vi "Main.vi"() -> ()   [LabVIEW 2019, in "gRPC Template Creation Utility.lvlib"]
uses:
  gRPC Template Creation Utility.lvlib
  TypeDefs/Project Settings.ctl
panel:
  in  "Library Suffix":string caption="Generated Library Suffix (\"_server\" / \"_client\" will be auto appended by default)"
  in  "Proto File Path":path[](array[path])
  in  "Generate":enum16{"gRPC Server", "gRPC Client", "Both"}(ring)
  in  "Target Name":string
  in  "Generated Library Name":string
  in  "Target Project":path
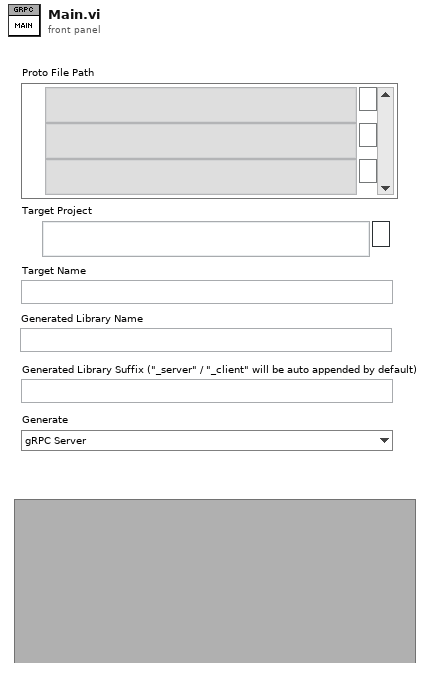
[diagram p1: front panel]
types:
  T1 = typedef "gRPC Template Creation Utility.lvlib/RPC Method Parameters.ctl" = cluster{"RPC Method Name":string, "Request Metadata Name":string, "Response Metadata Name":string, "Client Streaming":bool, "Server Streaming":bool}
  T2 = typedef "gRPC Template Creation Utility.lvlib/Message Metadata (Scripting).ctl" = cluster{"Version":i32, "Name":string, "Type Url":string, "Elements":T3[]}
  T3 = typedef "gRPC Template Creation Utility.lvlib/Message Element Metadata (Scripting).ctl" = cluster{"Field Name":string, "Embedded Message Name":string, "Protobuf Index":i32, "MessageElementType":T4, "Repeated":bool}
  T4 = typedef "gRPC Template Creation Utility.lvlib/Message Element Type.ctl" = enum32{"Int32Value", "FloatValue", "DoubleValue", "BoolValue", "StringValue", "MessageValue", "Int64Value", "UInt32Value", "UInt64Value", "EnumValue", "Bytes", "Fixed64", "Fixed32", "SFixed64", "SFixed32", "SInt64", "SInt32"}
  T5 = typedef "gRPC Template Creation Utility.lvlib/Project Settings.ctl" = cluster{"Target Project Path":path, "Target Name":string, "Server Name":string, "Library Path":path}
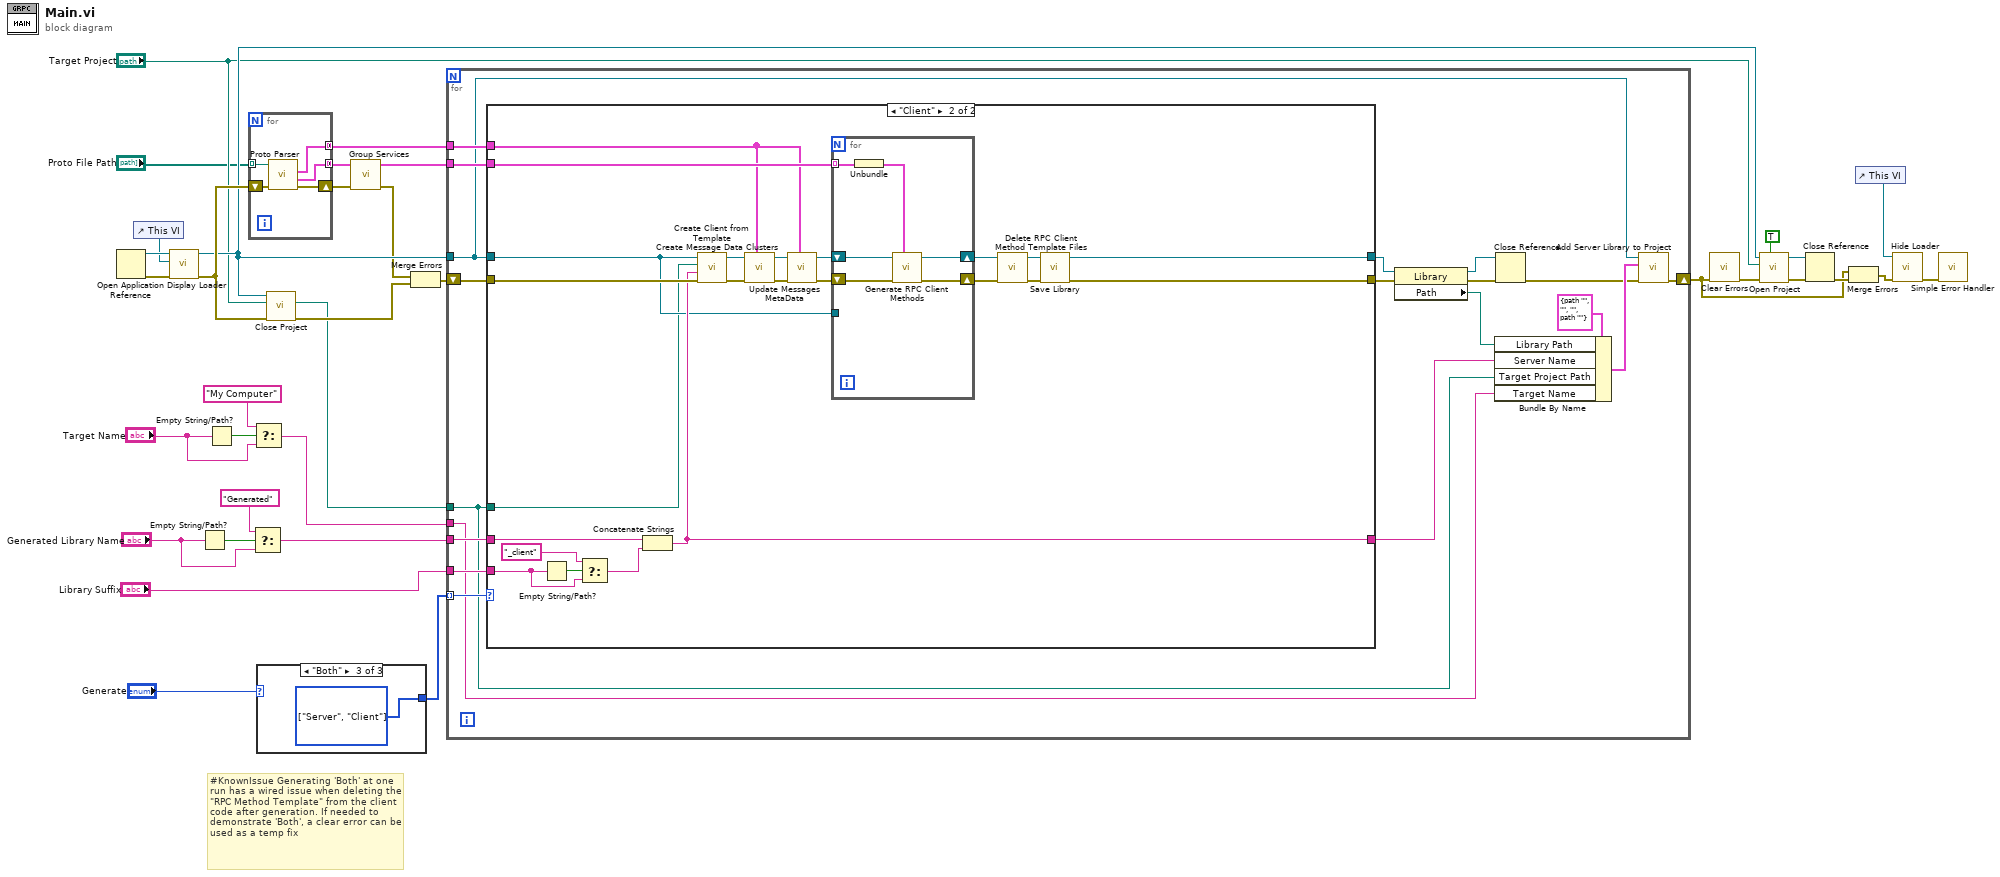
[diagram p0: block diagram]
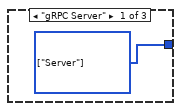
[diagram p2: hidden frame]
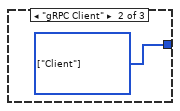
[diagram p3: hidden frame]
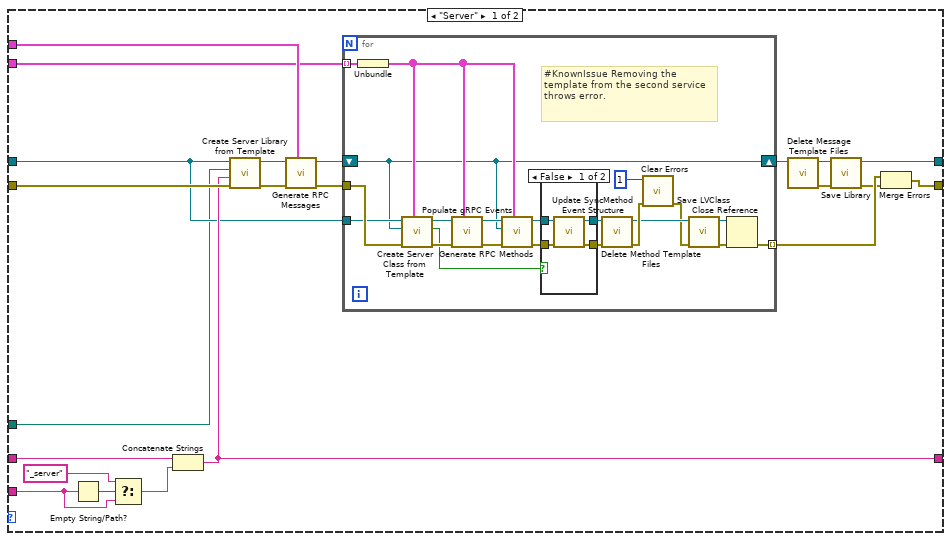
[diagram p4: hidden frame]
diagram:
  # "#KnownIssue Generating 'Both' at one run has a wired issue when deleting the \"RPC Method Template\" from the client code after generation. If needed to demonstrate 'Both', a clear error can be used as a temp fix"
  n1 = Open Application Reference() -> (0:w28:errorcluster, 3:w27:refnum<vi>)  [unwired: 4 in]
  n2 = control-ref of="This VI"() -> (w25:refnum<vi>)
  n3 = call "Display Loader.vi"("error in (no error)"=w28, "VI in"=w25, "application ref in"=w27) -> ("error out"=w26:errorcluster, "application ref out"=w13:refnum<vi>)  [unwired: 7 in]
  n4 = Empty String/Path?(string/path="Generated Library Name") -> (empty?=w35:bool)
  n5 = Empty String/Path?(string/path="Target Name") -> (empty?=w20:bool)
  n6 = for {
    tunnel: [w39] -> w30 mode=concatenating
    tunnel: [w38] -> w3 mode=concatenating
    shift-right: [w40] -> w5
    shift-left: w26 -> [w37]
    tunnel: "Proto File Path" -> [w36] mode=indexing
    n7 = call "Proto Parser.vi"("error in (no error)"=w37, ".proto file path"=w36) -> ("error out"=w40:errorcluster, "gRPC Method Parameters"=w38:T1[], "gRPC Messages Parameters"=w39:T2[])  [unwired: 7 in]
  }
  n8 = Select(t="Generated" ("Path"), s=w35, f="Generated Library Name") -> (s? t:f=w22:string)
  n9 = Select(t="My Computer" ("Path"), s=w20, f="Target Name") -> (s? t:f=w18:string)
  n10 = case shown="\"Both\"" "Generate" {
    tunnel: [w41 w42 w43] -> w17
    frame "gRPC Server" {
      w41 = enum16{"Server", "Client"}[] [enum."Server"] items=["Server", "Client"]
    }
    frame "gRPC Client" {
      w42 = enum16{"Server", "Client"}[] [enum."Client"] items=["Server", "Client"]
    }
    frame "Both" {
      w43 = enum16{"Server", "Client"}[] [enum."Server", enum."Client"] items=["Server", "Client"]
    }
  }
  n11 = call "Close Project.vi"("error in (no error)"=w26, "Project Path in"="Target Project", "Application reference"=w13) -> ("error out"=w32:errorcluster, "Project Path out"=w23:path)  [unwired: 6 in, 1 out]
  n12 = call "Group Services.vi"("error in"=w5, "gRPC Method Parameters"=w3) -> ("error out"=w4:errorcluster, "Service Methods"=w2:cluster{"gRPC Method Parameters":T1[]}[])  [unwired: 8 in]
  n13 = Merge Errors(w4, w32) -> (w31:errorcluster)
  n14 = for {
    tunnel: w30 -> [w61]
    tunnel: w2 -> [w60]
    tunnel: w23 -> [w45]
    tunnel: w22 -> [w53]
    tunnel: w18 -> [w44]
    tunnel: w13 -> [w51]
    shift-right: [w48] -> w7
    shift-left: w31 -> [w62]
    tunnel: w17 -> [w47] mode=indexing
    tunnel: "Library Suffix" -> [w46]
    n15 = case shown="\"Client\"" w47 {
      tunnel: w62 -> [w84 w134]
      tunnel: w61 -> [w83 w123]
      tunnel: w60 -> [w82 w133]
      tunnel: [w81 w132] -> w59
      tunnel: [w80 w120] -> w57
      tunnel: w53 -> [w79 w131]
      tunnel: [w78 w130] -> w52
      tunnel: w51 -> [w77 w129]
      tunnel: w45 -> [w76 w128]
      tunnel: w46 -> [w63 w113]
      frame "Server" {
        n16 = Empty String/Path?(string/path=w63) -> (empty?=w66:bool)
        n17 = Select(t="_server" ("string"), s=w66, f=w63) -> (s? t:f=w64:string)
        n18 = Concatenate Strings(w79, w64) -> (w78:string)
        n19 = call "Create Server Library from Template.vi"("error in (no error)"=w84, "Generated Server Name"=w78, "Target Project Path"=w76, "Application ref in"=w77) -> ("error out"=w74:errorcluster, "Server library out"=w75:refnum<vi>)  [unwired: 6 in]
        n20 = call "Generate RPC Messages.vi"("Messages MetaData"=w83, "error in (no error)"=w74, "Library"=w75) -> ("error out"=w72:errorcluster, "Library"=w73:refnum<vi>)  [unwired: 7 in]
        n21 = for {
          tunnel: w82 -> [w103] mode=indexing
          shift-right: [w94] -> w71
          shift-left: w73 -> [w94]
          tunnel: w77 -> [w104]
          tunnel: w72 -> [w105]
          tunnel: [w100] -> w70 mode=indexing
          # "#KnownIssue Removing the template from the second service throws error."
          n22 = Unbundle(w103) -> ("gRPC Method Parameters"=w95:T1[])
          n23 = call "Create Server Class from Template.vi"("gRPC Method Parameters"=w95, "error in (no error)"=w105, "Library"=w94, "Application ref in"=w104) -> ("error out"=w98:errorcluster, "Already Exists ?"=w89:bool, "LVClassLibrary in"=w99:refnum<vi>)  [unwired: 5 in]
          n24 = call "Populate gRPC Events.vi"("RPC Method Parameters"=w95, "error in (no error)"=w98, "Server class in"=w99) -> ("error out"=w96:errorcluster, "Server class out"=w97:refnum<vi>)  [unwired: 7 in]
          n25 = call "Generate RPC Methods.vi"("RPC Method Parameters"=w95, "error in (no error)"=w96, "Library"=w94, "Server class in"=w97) -> ("error out"=w91:errorcluster, "Server class out"=w93:refnum<vi>)  [unwired: 6 in]
          n26 = case shown="False" w89 {
            tunnel: w93 -> [w109 w111]
            tunnel: [w108 w111] -> w92
            tunnel: w91 -> [w107 w110]
            tunnel: [w106 w110] -> w90
            frame False {
              n27 = call "Update SyncMethod Event Structure.vi"("error in (no error)"=w107, "Server class in"=w109) -> ("error out"=w106:errorcluster, "Server class out"=w108:refnum<vi>)  [unwired: 8 in]
            }
            frame True {
            }
          }
          n28 = call "Delete Method Template Files.vi"("error in (no error)"=w90, "LVClassLibrary in"=w92) -> ("error out"=w87:errorcluster, "LVClassLibrary out"=w86:refnum<vi>)  [unwired: 8 in]
          n29 = call <vilib>:"Clear Errors.vi"("error in (no error)"=w87, "specific error code to clear (0: all)"=1) -> ("error out"=w85:errorcluster)  [unwired: 4 in, 1 out]
          n30 = call "Save LVClass.vi"("error in (no error)"=w85, "LVClassLibrary in"=w86) -> ("error out"=w102:errorcluster, "LVClassLibrary out"=w101:refnum<vi>)  [unwired: 8 in]
          n31 = Close Reference(reference=w101, error in (no error)=w102) -> (error out=w100:errorcluster)
        }
        n32 = call "Delete Message Template Files.vi"("Library"=w71) -> ("error out"=w69:errorcluster, "Library"=w67:refnum<vi>)  [unwired: 9 in]
        n33 = call "Save Library.vi"("error in (no error)"=w69, "Library in"=w67) -> ("error out"=w68:errorcluster, "Library out"=w81:refnum<vi>)  [unwired: 8 in]
        n34 = Merge Errors(w70, w68) -> (w80:errorcluster)
      }
      frame "Client" {
        n35 = Empty String/Path?(string/path=w113) -> (empty?=w115:bool)
        n36 = Select(t="_client" ("string"), s=w115, f=w113) -> (s? t:f=w112:string)
        n37 = Concatenate Strings(w131, w112) -> (w130:string)
        n38 = call "Create Client from Template.vi"("error in (no error)"=w134, "Generated Server Name"=w130, "Target Project Path"=w128, "Application ref in"=w129) -> ("error out"=w127:errorcluster, "Server library out"=w126:refnum<vi>)  [unwired: 6 in]
        n39 = call "Create Message Data Clusters.vi"("Message parameters"=w123, "error in (no error)"=w127, "Library"=w126) -> ("error out"=w125:errorcluster, "Library"=w124:refnum<vi>)  [unwired: 7 in]
        n40 = call "Update Messages MetaData.vi"("Messages MetaData"=w123, "error in (no error)"=w125, "Library"=w124) -> ("error out"=w122:errorcluster, "Library"=w121:refnum<vi>)  [unwired: 7 in]
        n41 = for {
          tunnel: w133 -> [w140] mode=indexing
          shift-right: [w135] -> w119
          shift-left: w121 -> [w137]
          tunnel: w129 -> [_]
          shift-right: [w136] -> w116
          shift-left: w122 -> [w138]
          n42 = Unbundle(w140) -> ("gRPC Method Parameters"=w139:T1[])
          n43 = call "Generate RPC Client Methods.vi"("RPC Method Parameters"=w139, "error in (no error)"=w138, "Library"=w137) -> ("error out"=w136:errorcluster, "Library"=w135:refnum<vi>)  [unwired: 7 in]
        }
        n44 = call "Delete RPC Client Method Template Files.vi"("error in (no error)"=w116, "Library"=w119) -> ("error out"=w117:errorcluster, "Library"=w118:refnum<vi>)  [unwired: 8 in]
        n45 = call "Save Library.vi"("error in (no error)"=w117, "Library in"=w118) -> ("error out"=w120:errorcluster, "Library out"=w132:refnum<vi>)  [unwired: 8 in]
      }
    }
    n46 = property class="Library"(reference=w59, error in=w57) -> (reference out=w58:refnum<vi>, error out=w50:errorcluster, "Path"=w55:path)
    n47 = Bundle By Name(cluster=T5 {"Target Project Path"=path "", "Target Name"="", "Server Name"="", "Library Path"=path ""} ("Project Settings"), "Library Path"=w55, "Server Name"=w52, "Target Project Path"=w45, "Target Name"=w44) -> (w54:T5)
    n48 = Close Reference(reference=w58, error in (no error)=w50) -> (error out=w49:errorcluster)
    n49 = call "Add Server Library to Project.vi"("error in (no error)"=w49, "Project Settings"=w54, "Application in"=w51) -> ("error out"=w48:errorcluster)  [unwired: 8 in]
  }
  n50 = call <vilib>:"Clear Errors.vi"("error in (no error)"=w7) -> ("error out"=w9:errorcluster)  [unwired: 5 in, 1 out]
  n51 = call "Open Project.vi"("Open Project Window ?"=TRUE, "error in (no error)"=w9, "Project Path in"="Target Project", "Application reference"=w13) -> ("error out"=w11:errorcluster, "Application out"=w12:refnum<vi>)  [unwired: 5 in, 1 out]
  n52 = Close Reference(reference=w12, error in (no error)=w11) -> (error out=w15:errorcluster)
  n53 = Merge Errors(w7, w15) -> (w8:errorcluster)
  n54 = control-ref of="This VI"() -> (w29:refnum<vi>)
  n55 = call "Hide Loader.vi"("error in (no error)"=w8, "VI in"=w29) -> ("error out"=w24:errorcluster)  [unwired: 9 in]
  n56 = call <vilib>:"Simple Error Handler.vi"("error in (no error)"=w24) -> ()  [unwired: 4 in, 5 out]
